vi "Broadcast Item Key.vi"(3 "status":string="status", 4 "target":string="target", 5 "source":string="source") -> (2 "key":string="status@source->target")   [LabVIEW 2020, in "Communicable State Machine.lvlib" / "BroadcastRegistry.lvclass"]
uses:
  BroadcastRegistry.lvclass
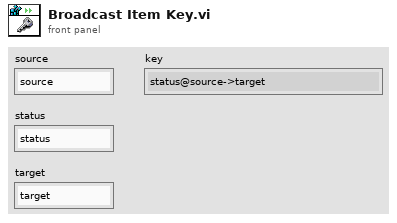
[diagram p1: front panel]
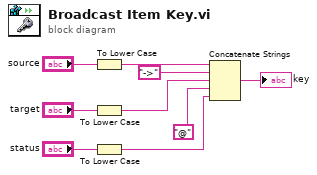
[diagram p0: block diagram]
diagram:
  n1 = To Lower Case(string="source") -> (all lower case string=w8:string)
  n2 = To Lower Case(string="target") -> (all lower case string=w3:string)
  n3 = To Lower Case(string="status") -> (all lower case string=w1:string)
  n4 = Concatenate Strings(w8, "->" ("string"), w3, "@" ("string"), w1) -> (→"key":string)
